vi "Store Built Enum.vi"(6 "Built Enumeration":T1, 8 "error in (no error)":errorcluster, 11 "LV-Protoc in":refnum<class "LV-Protoc.lvclass">) -> (0 "error out":errorcluster, 3 "LV-Protoc out":refnum<class "LV-Protoc.lvclass">)   [LabVIEW 2020, in "LV-Protoc.lvlib" / "LV-Protoc.lvclass"]
uses:
  LV-Protoc.lvclass
  Enumeration Paths.ctl
  LV-Protoc.lvclass/LV-Protoc.ctl
  LV-Protoc.lvlib
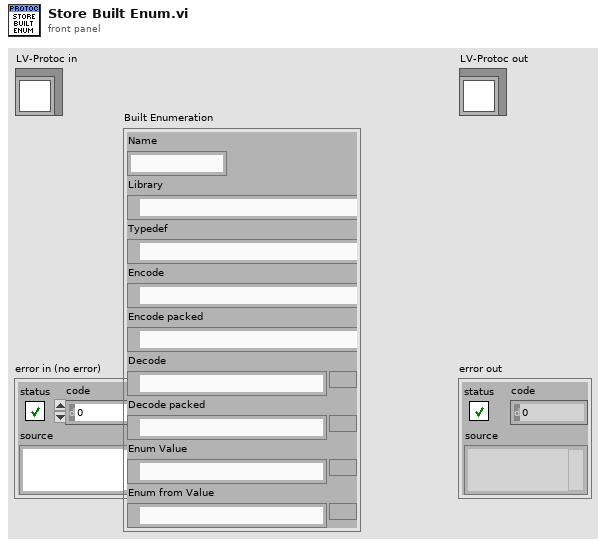
[diagram p1: front panel]
types:
  T1 = typedef "LV-Protoc.lvlib/Enumeration Paths.ctl" = cluster{"Name":string, "Library":path, "Typedef":path, "Encode":path, "Encode packed":path, "Decode":path, "Decode packed":path, "Enum Value":path, "Enum from Value":path}
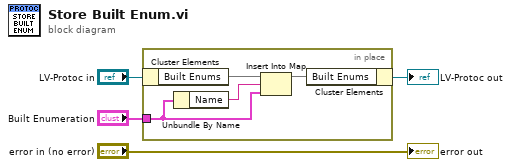
[diagram p0: block diagram]
diagram:
  n1 = in-place {
    in-place-border: "Built Enumeration" -> [w6]
    n2 = in-place-cluster #1("LV-Protoc in") -> ("Built Enums"=w8:map{string, T1})
    n3 = Unbundle By Name(w6) -> ("Name"=w7:string)
    n4 = Insert Into Map(map in=w8, key=w7, value=w6) -> (map out=w5:map{string, T1})  [unwired: 2 out]
    n5 = in-place-cluster #1("Built Enums"=w5) -> (→"LV-Protoc out":refnum<class "LV-Protoc.lvclass">)
  }
  "error out" <- "error in (no error)"
